vi "Write value 1.vi"(8 "error in (no error)":errorcluster, 10 "value 1":dbl, 11 "DataLogging in":refnum<class "DataLogging.lvclass">) -> (0 "error out":errorcluster, 3 "DataLogging out":refnum<class "DataLogging.lvclass">)   [LabVIEW 2017, in "DataLogging.lvclass"]
uses:
  DataLogging.lvclass
  DataLogging.lvclass/DataLogging.ctl
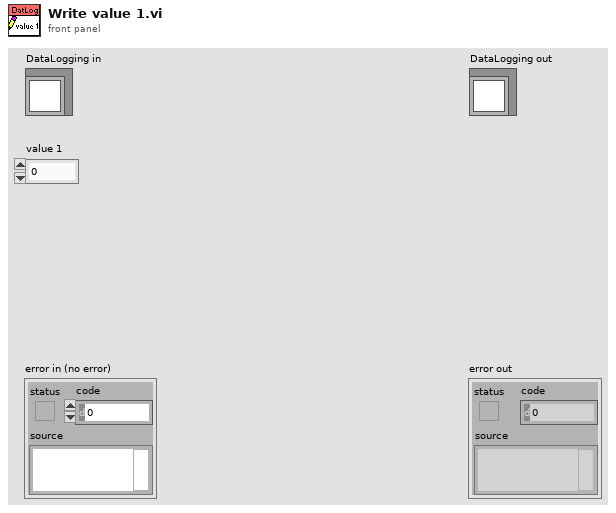
[diagram p1: front panel]
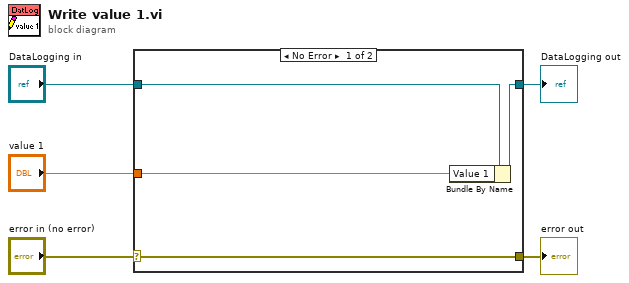
[diagram p0: block diagram]
diagram:
  n1 = case shown="No Error" "error in (no error)" {
    selector: "error in (no error)" -> [w9 w10]
    tunnel: [w9 w10] -> w4
    tunnel: [w7 w11] -> w2
    tunnel: "DataLogging in" -> [w8 w11]
    tunnel: "value 1" -> [w6 _]
    frame No Error {
      n2 = Bundle By Name(cluster=w8, "Value 1"=w6) -> (w7:refnum<class "DataLogging.lvclass">)
    }
    frame Error {
    }
  }
  "error out" <- w4
  "DataLogging out" <- w2
